vi "FX1E.vi"(11 "Variables and Memory in":T1 {"GFX" format="%02x"}) -> (3 "Variables and Memory out":T1 {"GFX" format="%02x"})   [LabVIEW 2021]
uses:
  Controls/ClusterF.ctl
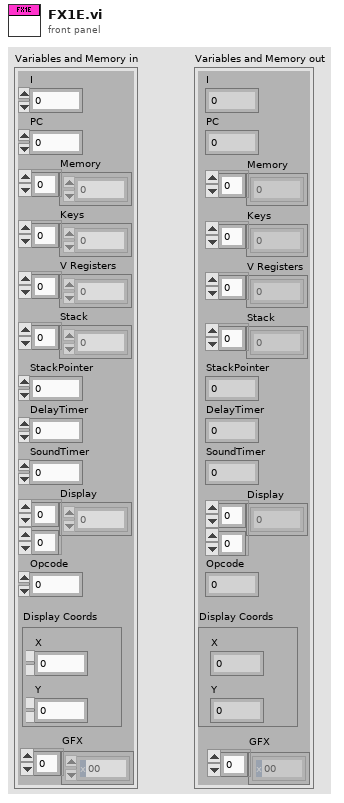
[diagram p1: front panel]
types:
  T1 = typedef "ClusterF.ctl" = cluster{"I":u16, "PC":u16, "Memory":u8[], "Keys":u8[], "V Registers":u8[], "Stack":u16[], "StackPointer":u16, "DelayTimer":u8, "SoundTimer":u8, "Display":u8[][], "Opcode":u16, "Display Coords":cluster{"X":u8, "Y":u8}, "GFX":u8[]}
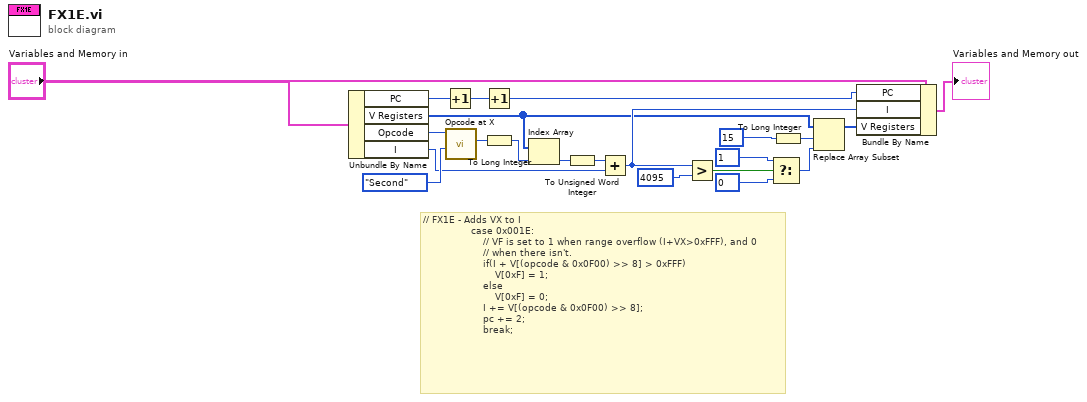
[diagram p0: block diagram]
diagram:
  # "// FX1E - Adds VX to I\n                case 0x001E:\n                    // VF is set to 1 when range overflow (I+VX>0xFFF), and 0\n                    // when there isn't.\n                    if(I + V[(opcode & 0x0F00) >> 8] > 0xFFF)\n                        V[0xF] = 1;\n                    else\n                        V[0xF] = 0;\n                    I += V[(opcode & 0x0F00) >> 8];\n                    pc += 2;\n                    break;"
  n1 = Unbundle By Name("Variables and Memory in") -> ("PC"=w2:u16, "V Registers"=w13:u8[], "Opcode"=w10:u16, "I"=w7:u16)
  n2 = Increment(x=w2) -> (x+1=w1:u16)
  n3 = call "Opcode at X.vi"("X Position"=enum16{"First", "Second", "Third", "Fourth"}."Second", "Opcode"=w10) -> ("Opcode at X Position (U8)"=w9:u8)  [unwired: 9 in]
  n4 = Increment(x=w1) -> (x+1=w5:u16)
  n5 = To Long Integer(number=w9) -> (32bit integer=w11:i32)
  n6 = Index Array(array=w13, index=w11) -> (element=w6:u8)
  n7 = To Unsigned Word Integer(number=w6) -> (unsigned 16bit integer=w12:u16)
  n8 = Add(x=w12, y=w7) -> (x+y=w16:u16)
  n9 = Greater?(x=w16, y=u16 4095) -> (0:w17:bool)
  n10 = Select(t=u8 1, s=w17, f=u8 0) -> (s? t:f=w18:u8)
  n11 = To Long Integer(number=u8 15) -> (32bit integer=w15:i32)
  n12 = Replace Array Subset(array=w13, new element=w18, index=w15) -> (w21:u8[])
  n13 = Bundle By Name(cluster="Variables and Memory in", "PC"=w5, "I"=w16, "V Registers"=w21) -> (→"Variables and Memory out":T1)
